vi "Read Geodes.vi"(11 "Mine in":refnum<class "Mine.lvclass">) -> (2 "Geodes":u8, 3 "Mine out":refnum<class "Mine.lvclass">)   [LabVIEW 2023, in "d19.lvlib" / "Mine.lvclass"]
uses:
  Mine.lvclass
  Mine.lvclass/Mine.ctl
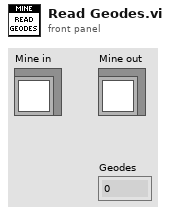
[diagram p1: front panel]
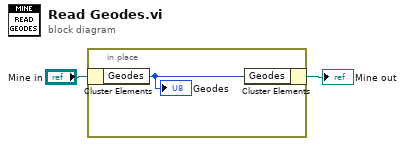
[diagram p0: block diagram]
diagram:
  n1 = in-place {
    n2 = in-place-cluster #1("Mine in") -> ("Geodes"=w3:u8)
    "Geodes" <- w3
    n3 = in-place-cluster #1("Geodes"=w3) -> (→"Mine out":refnum<class "Mine.lvclass">)
  }
